vi "Save_Data.vi"(2 "error in (no error)":errorcluster, 3 "History Data":T1) -> (0 "error out":errorcluster)   [LabVIEW 2021]
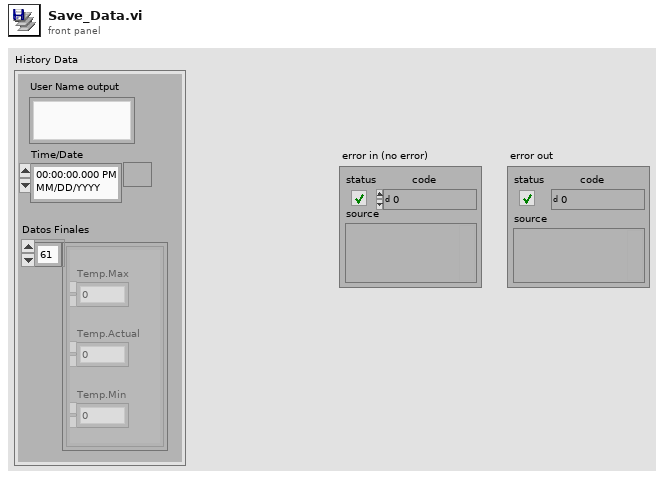
[diagram p1: front panel]
types:
  T1 = cluster{"User Name output":string, "Time/Date":timestamp, "Datos Finales":cluster{"Temp.Max":dbl, "Temp.Actual":dbl, "Temp.Min":dbl}[]}
  T2 = enum16{"open", "replace", "create", "open or create", "replace or create", "replace or create with confirmation"}
  T3 = cluster{"Temp.Max":dbl, "Temp.Actual":dbl, "Temp.Min":dbl}[]
  T4 = cluster{"Temp.Max":dbl, "Temp.Actual":dbl, "Temp.Min":dbl}
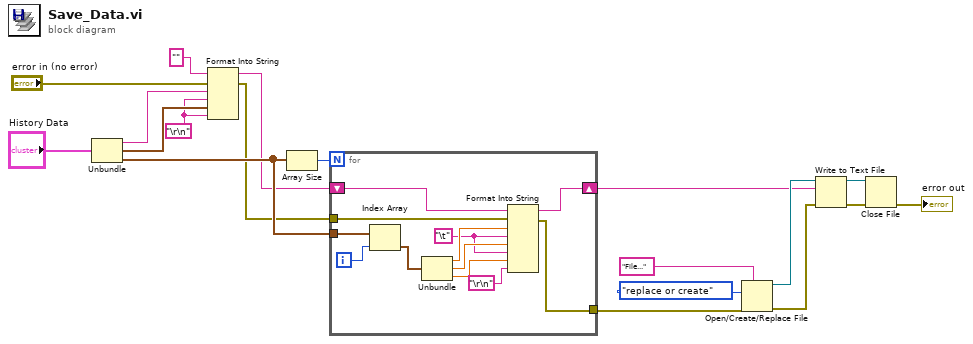
[diagram p0: block diagram]
diagram:
  w6 = "\r\n"
  n1 = Unbundle("History Data") -> ("User Name output"=w8:string, "Time/Date"=w7:timestamp, "Datos Finales"=w9:T3)
  n2 = Format Into String(initial string="", error in="error in (no error)", w8, w6, w7, w6) -> (resulting string=w5:string, error out=w2:errorcluster)  [unwired: 1 in]
  n3 = Array Size(array=w9) -> (size(s)=w19:i32)
  n4 = for {
    N: w19 -> [_]
    tunnel: w9 -> [w31]
    shift-right: [w23] -> w12
    shift-left: w5 -> [w22]
    tunnel: w2 -> [w21]
    tunnel: [w20] -> w1
    i -> [w30]
    w25 = "\t"
    n5 = Index Array(array=w31, index=w30) -> (element=w29:T4)
    n6 = Unbundle(w29) -> ("Temp.Max"=w28:dbl, "Temp.Actual"=w27:dbl, "Temp.Min"=w26:dbl)
    n7 = Format Into String(initial string=w22, error in=w21, w28, w25, w27, w25, w26, "\r\n") -> (resulting string=w23:string, error out=w20:errorcluster)  [unwired: 1 in]
  }
  n8 = Open/Create/Replace File(error in=w1, prompt="File...", operation (0:open)=T2."replace or create") -> (refnum out=w15:refnum<file>, error out=w18:errorcluster)  [unwired: 3 in, 1 out]
  n9 = Write to Text File(file (use dialog)=w15, text=w12, error in=w18) -> (refnum out=w16:refnum<file>, error out=w17:errorcluster)  [unwired: 1 in, 1 out]
  n10 = Close File(refnum=w16, error in=w17) -> (error out=→"error out":errorcluster)  [unwired: 1 out]
